vi "ChicagoStyleCheesePizza.vi"(8 "error in (no error)":errorcluster) -> (0 "error out":errorcluster, 3 "ChicagoStyleCheesePizza":refnum<class "ChicagoStyleCheesePizza.lvclass">)   [LabVIEW 2020, in "FactoryMethod.lvlib" / "PizzaFactoryMethod.lvlib" / "ChicagoStyleCheesePizza.lvclass"]
uses:
  ChicagoStyleCheesePizza.lvclass
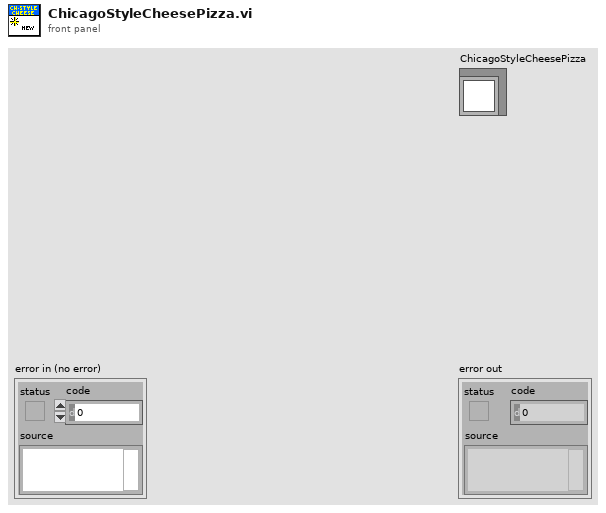
[diagram p1: front panel]
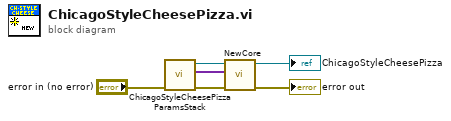
[diagram p0: block diagram]
diagram:
  n1 = call "ChicagoStyleCheesePizzaParamsStack.vi"("error iN"="error in (no error)") -> ("error out"=w6:errorcluster, "HierarchyParams"=w5:variant[], "ChicagoStyleCheesePizza"=w1:refnum<class "ChicagoStyleCheesePizza.lvclass">)  [unwired: 8 in]
  n2 = call-dynamic "NewCore.vi"("error in (no error)"=w6, "ParamsArray"=w5, "ChicagoStyleCheesePizza"=w1) -> ("error out"=→"error out":errorcluster, "ChicagoStyleCheesePizza"=→"ChicagoStyleCheesePizza":refnum<class "ChicagoStyleCheesePizza.lvclass">)  [unwired: 7 in]
